vi "Add JSONtext to palette.vi"   [LabVIEW 2017]
uses:
  <vilib>/Palette API/Palette Menu/Public Type Define/Palette type.ctl
  <vilib>/Palette API/Palette Menu/Public Type Define/Item.ctl
  <vilib>/Palette API/Palette Menu/Palette Menu.lvlib
types:
  T1 = typedef "Palette Menu.lvlib/Item.ctl" = cluster{"item path":path, "library path (.lvlib)":path, "use default lvlib palette":bool, "short name":string, "place VI contents":bool, "hide synchronized item":bool, "reserve spot for synch item":bool, "configure when placing VI contents":bool}
  T2 = typedef "Palette Menu.lvlib/Palette type.ctl" = i32
  T3 = typedef "Palette Menu.lvlib/Palette Data.ctl" = cluster{"display name":string, "view format":T4, "palette width":i16, "items":T5, "256 color icon":picture, "B&W color icon":picture, "help information":T6, "palette description":string, "synchronize information":T7}
  T4 = typedef "Palette Menu.lvlib/View Format.ctl" = u16
  T5 = typedef "Palette Menu.lvlib/Items.ctl" = T1[]
  T6 = typedef "Palette Menu.lvlib/Help Info.ctl" = cluster{"help tag":string, "help file path ":path}
  T7 = typedef "Palette Menu.lvlib/Synchronize Info.ctl" = cluster{"synchronize with directory":bool, "synchronize directory path":path}
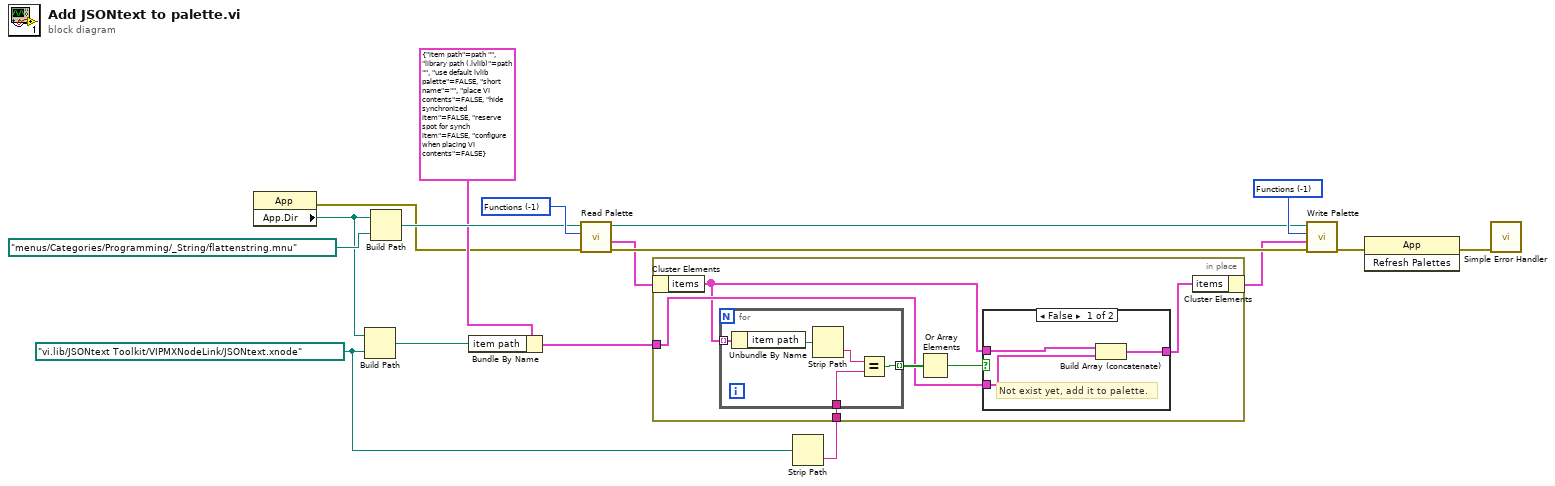
[diagram p0: block diagram]
diagram:
  w2 = path "vi.lib/JSONtext Toolkit/VIPMXNodeLink/JSONtext.xnode"
  w12 = T2 -1 items=["Functions"=-1, "Controls"=-2] ("palette type")
  w15 = T2 -1 items=["Functions"=-1, "Controls"=-2] ("palette type")
  n1 = property class="App"() -> (error out=w3:errorcluster, "App.Dir"=w4:path)  [unwired: 2 in, 1 out]
  n2 = Build Path(base path=w4, name or relative path=w2) -> (appended path=w8:path)
  n3 = Build Path(base path=w4, name or relative path=path "menus/Categories/Programming/_String/flattenstring.mnu") -> (appended path=w10:path)
  n4 = Bundle By Name(cluster=T1 {"item path"=path "", "library path (.lvlib)"=path "", "use default lvlib palette"=FALSE, "short name"="", "place VI contents"=FALSE, "hide synchronized item"=FALSE, "reserve spot for synch item"=FALSE, "configure when placing VI contents"=FALSE} ("Items"), "item path"=w8) -> (w7:T1)
  n5 = call <vilib>:"Read Palette.vi"("error in (no error)"=w3, "palette type"=w12, "palette path"=w10) -> ("error out"=w14:errorcluster, "palette data"=w6:T3, "duplicate palette path"=w13:path)  [unwired: 1 in, 5 out]
  n6 = Strip Path(path=w2) -> (name=w1:string)  [unwired: 1 out]
  n7 = in-place {
    in-place-border: w7 -> [w20]
    in-place-border: w1 -> [w23]
    n8 = in-place-cluster #1(w6) -> ("items"=w18:T5)
    n9 = for {
      tunnel: w18 -> [w32] mode=indexing
      tunnel: w23 -> [w29]
      tunnel: [w28] -> w22 mode=indexing
      n10 = Unbundle By Name(w32) -> ("item path"=w31:path)
      n11 = Strip Path(path=w31) -> (name=w30:string)  [unwired: 1 out]
      n12 = Equal?(x=w30, y=w29) -> (x = y?=w28:bool)
    }
    n13 = Or Array Elements(Boolean array=w22) -> (logical OR=w21:bool)
    n14 = case shown="False" w21 {
      tunnel: w20 -> [w26 _]
      tunnel: [w25 w27] -> w19
      tunnel: w18 -> [w24 w27]
      frame False {
        # "Not exist yet, add it to palette."
        n15 = Build Array (concatenate)(w24, w26) -> (w25:T5)
      }
      frame True {
        # "Alreay exists on palette,\ndo nothing."
      }
    }
    n16 = in-place-cluster #1("items"=w19) -> (w5:T3)
  }
  n17 = call <vilib>:"Write Palette.vi"("error in (no error)"=w14, "palette data"=w5, "palette type"=w15, "palette path"=w13) -> ("error out"=w17:errorcluster)  [unwired: 1 in, 6 out]
  n18 = invoke class="App" method="Refresh Palettes"(error in=w17) -> (error out=w16:errorcluster)  [unwired: 2 in, 2 out]
  n19 = call <vilib>:"Simple Error Handler.vi"("error in (no error)"=w16) -> ()  [unwired: 1 in, 8 out]
